vi "Registry For Assert VIs.vi"() -> ()   [LabVIEW 2013, in "Caraya.lvlib" / "Assert.lvclass"]
uses:
  Assert.lvclass
panel:
  in  "registry":string[](array[string])
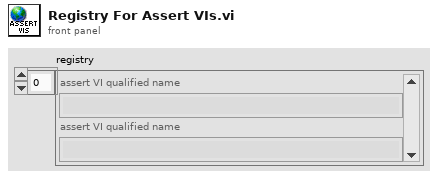
[diagram p1: front panel]
diagram:
